vi "VCL_2_DSC_BATCH.vi"(8 "error in (no error)":errorcluster, 11 "path to logfile or directory":path) -> (0 "error out":errorcluster)   [LabVIEW 2016, in "VCL_2_DSC.lvclass"]
uses:
  VCL_2_DSC.lvclass
  <vilib>/addons/WireFlow/_WF_ProgressBar.llb/ProgressBar_WireFlow.lvclass
panel:
  in  "Write to DSC?":bool
  out "standard output":string
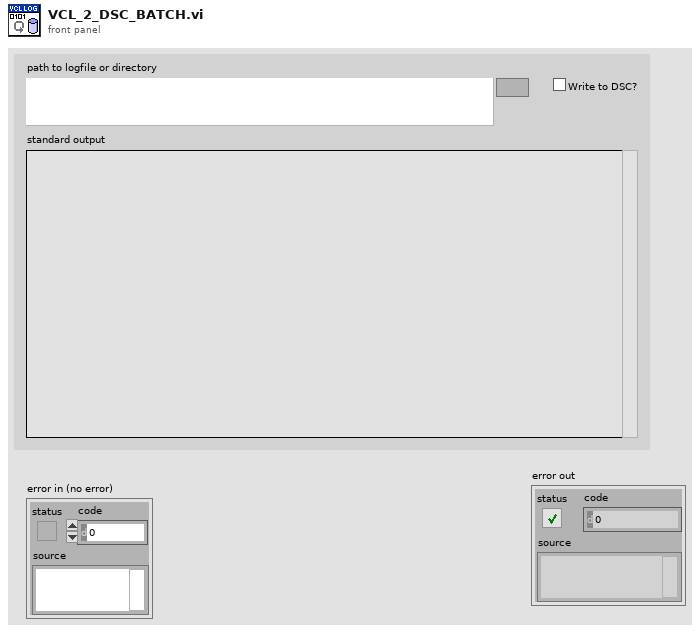
[diagram p1: front panel]
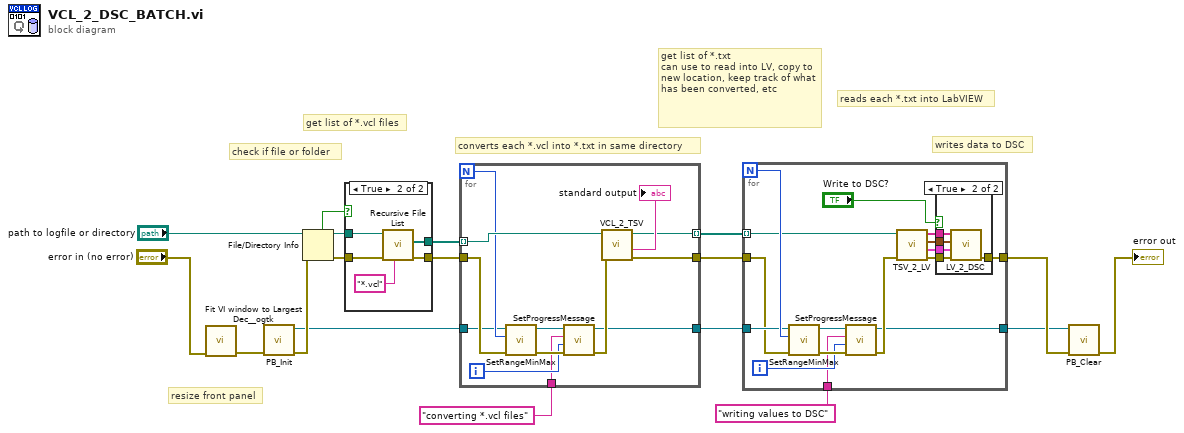
[diagram p0: block diagram]
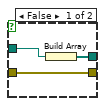
[diagram p3: hidden frame]
diagram:
  # "writes data to DSC"
  # "get list of *.txt\ncan use to read into LV, copy to new location, keep track of what has been converted, etc"
  # "reads each *.txt into LabVIEW"
  # "converts each *.vcl into *.txt in same directory"
  # "resize front panel"
  # "check if file or folder"
  # "get list of *.vcl files"
  n1 = call <userlib>:"Fit VI window to Largest Dec__ogtk.vi"("error in (no error)"="error in (no error)") -> ("error out"=w11:errorcluster)  [unwired: 5 in, 1 out]
  n2 = call <vilib>:"PB_Init.vi"("error in (no error)"=w11) -> ("error out"=w12:errorcluster, "WF-ProgressBar out"=w9:refnum<class "ProgressBar_WireFlow.lvclass">)  [unwired: 9 in]
  n3 = File/Directory Info(path="path to logfile or directory", error in=w12) -> (path out=w13:path, directory=w15:bool, error out=w16:errorcluster)  [unwired: 4 out]
  n4 = case shown="True" w15 {
    tunnel: [w19 w26] -> w18
    tunnel: [w20 w25] -> w17
    tunnel: w16 -> [w19 w24]
    tunnel: w13 -> [w21 w23]
    frame False {
      n5 = Build Array(w21) -> (w20:path[])
    }
    frame True {
      n6 = call <vilib>:"Recursive File List.vi"("pattern"="*.vcl", "error in (no error)"=w24, "Folder Path"=w23) -> ("error out"=w26:errorcluster, "All Files in Dir"=w25:path[])  [unwired: 4 in, 3 out]
    }
  }
  n7 = for {
    N -> [w36]
    tunnel: w18 -> [w37]
    tunnel: w17 -> [w38] mode=indexing
    tunnel: w9 -> [w35]
    tunnel: [w30] -> w8
    tunnel: "converting *.vcl files" ("Message") -> [w29]
    tunnel: [w28] -> w2 mode=indexing
    tunnel: [w27] -> w1
    i -> [w33]
    n8 = call-dynamic "SetRangeMinMax.vi"("error in (no error)"=w37, "Max (1)"=w36, "WF-ProgressBar in"=w35) -> ("error out"=w34:errorcluster, "WF-ProgressBar out"=w32:refnum<class "ProgressBar_WireFlow.lvclass">)  [unwired: 7 in]
    n9 = call-dynamic "SetProgressMessage.vi"("error in (no error)"=w34, "Progress value (NaN no update)"=w33, "Message"=w29, "WF-ProgressBar in"=w32) -> ("error out"=w31:errorcluster, "WF-ProgressBar out"=w30:refnum<class "ProgressBar_WireFlow.lvclass">)  [unwired: 5 in, 1 out]
    n10 = call "VCL_2_TSV.vi"("error in (no error)"=w31, "Path to VCL file"=w38) -> ("error out"=w27:errorcluster, "standard output"=→"standard output":string, "path to txt file"=w28:path)  [unwired: 7 in]
  }
  n11 = for {
    N -> [w48]
    tunnel: w8 -> [w47]
    tunnel: [w44] -> w6
    tunnel: "writing values to DSC" ("Message") -> [w42]
    tunnel: w2 -> [w41] mode=indexing
    tunnel: w1 -> [w46]
    tunnel: [w51] -> w7
    i -> [w43]
    n12 = call-dynamic "SetRangeMinMax.vi"("error in (no error)"=w46, "Max (1)"=w48, "WF-ProgressBar in"=w47) -> ("error out"=w49:errorcluster, "WF-ProgressBar out"=w50:refnum<class "ProgressBar_WireFlow.lvclass">)  [unwired: 7 in]
    n13 = call-dynamic "SetProgressMessage.vi"("error in (no error)"=w49, "Progress value (NaN no update)"=w43, "Message"=w42, "WF-ProgressBar in"=w50) -> ("error out"=w45:errorcluster, "WF-ProgressBar out"=w44:refnum<class "ProgressBar_WireFlow.lvclass">)  [unwired: 5 in, 1 out]
    n14 = call "TSV_2_LV.vi"("error in (no error)"=w45, "tsv file path (dialog if empty)"=w41) -> ("error out"=w55:errorcluster, "Data Array"=w54:cluster{dbl[]}[], "Time Array (common)"=w53:timestamp[], "Name Array"=w52:string[])  [unwired: 6 in]
    n15 = case shown="True" "Write to DSC?" {
      tunnel: w55 -> [w56 w61]
      tunnel: w54 -> [_ w60]
      tunnel: w53 -> [_ w59]
      tunnel: w52 -> [_ w58]
      tunnel: [w56 w57] -> w51
      frame False {
      }
      frame True {
        n16 = call "LV_2_DSC.vi"("error in (no error)"=w61, "Data Array"=w60, "Time Array (common)"=w59, "Name Array"=w58) -> ("error out"=w57:errorcluster)  [unwired: 7 in]
      }
    }
  }
  n17 = call-dynamic "PB_Clear.vi"("error in (no error)"=w7, "WF-ProgressBar in"=w6) -> ("error out"=→"error out":errorcluster)  [unwired: 8 in, 1 out]
